vi "Thermocouple.vi"() -> ()   [LabVIEW 2020]
uses:
  <vilib>/Analysis/baseanly.llb/Mean (DBL).vi
  Globals.vi
  <vilib>/Analysis/NI_AALBase.lvlib
panel:
  out "Thermometer":dbl(slide) scale=0.0..100.0
  in  "stop (F)":bool
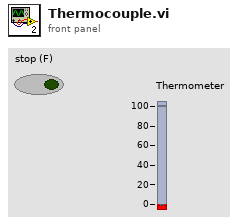
[diagram p1: front panel]
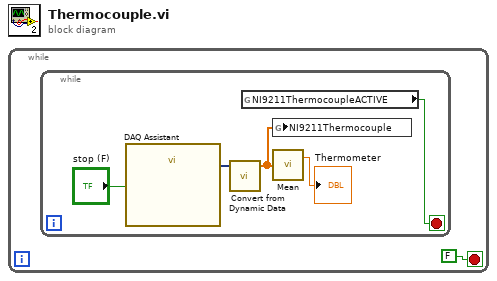
[diagram p0: block diagram]
diagram:
  n1 = while {
    stop <- FALSE stop-if-true
    n2 = while {
      stop <- w2 stop-if-true
      n3 = call "DAQ Assistant"("stop (F)"="stop (F)") -> ("data"=w5:dynamicdata)  [unwired: 15 in, 3 out]
      n4 = call "Convert from Dynamic Data"("Dynamic Data Type"=w5) -> ("Array"=w3:dbl[])  [unwired: 3 in]
      n5 = global read "Globals.vi" "NI9211ThermocoupleACTIVE"() -> (w2:bool)
      n6 = global write "Globals.vi" "NI9211Thermocouple"(w3) -> ()
      n7 = call-poly <vilib>:"Mean.vi"("X"=w3) -> ("mean"=→"Thermometer":dbl)  [unwired: 1 out]
    }
  }
